vi "Get Device SN.vi"(8 "error in (no error)":errorcluster) -> (0 "error out":errorcluster, 2 "SN":string)   [LabVIEW 2018]
doc: "Returns MAC address on Windows, and device SN on RT Linux. Keeps the value in a shift register for future use."
uses:
  <vilib>/nisyscfg/nisyscfg.lvlib
  <resource>/objmgr/nisysapi.rc
  <vilib>/nisyscfg/Close (System).vi
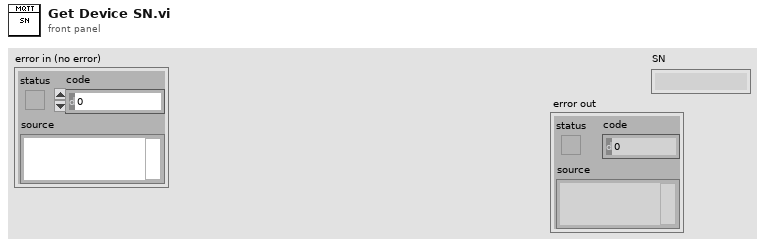
[diagram p1: front panel]
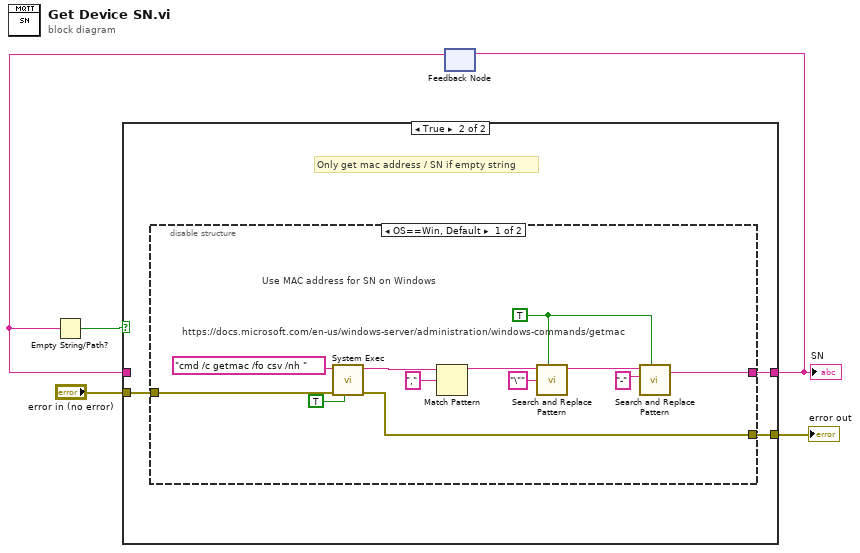
[diagram p0: block diagram]
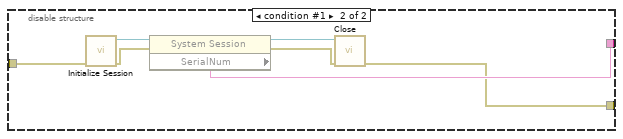
[diagram p3: hidden frame]
diagram:
  n1 = feedback #1() -> (w2:string)  [unwired: 1 in]
  n2 = Empty String/Path?(string/path=w2) -> (empty?=w1:bool)
  n3 = case shown="True" w1 {
    tunnel: [w6 w10] -> w3
    tunnel: [w7 w9] -> w5
    tunnel: "error in (no error)" -> [w7 w8]
    tunnel: w2 -> [w6 _]
    frame False {
    }
    frame True {
      # "Only get mac address / SN if empty string"
      n4 = disable-structure shown="OS==Win, Default" {
        disable-tunnel: [w13 w28] -> w10
        disable-tunnel: [w12 w24] -> w9
        disable-tunnel: w8 -> [w11 w23]
        frame condition #0 (active) {
          w15 = TRUE ("replace all? (F)")
          # "Use MAC address for SN on Windows"
          # "https://docs.microsoft.com/en-us/windows-server/administration/windows-commands/getmac"
          n5 = call <vilib>:"System Exec.vi"("run minimized? (F)"=TRUE, "error in (no error)"=w11, "command line"="cmd /c getmac /fo csv /nh ") -> ("error out"=w12:errorcluster, "standard output"=w20:string)  [unwired: 5 in, 2 out]
          n6 = Match Pattern(string=w20, regular expression="," ("delimiter (Tab)")) -> (before substring=w18:string)  [unwired: 1 in, 3 out]
          n7 = call <vilib>:"Search and Replace Pattern.vi"("string"=w18, "regular expression (\"\")"="\"" ("regular expression (\"\")"), "replace all? (F)"=w15) -> ("result string"=w14:string)  [unwired: 2 in, 1 out]
          n8 = call <vilib>:"Search and Replace Pattern.vi"("string"=w14, "regular expression (\"\")"="-" ("regular expression (\"\")"), "replace all? (F)"=w15) -> ("result string"=w13:string)  [unwired: 2 in, 1 out]
        }
        frame condition #1 {
          n9 = call <vilib>:"Initialize Session.vi"("error in (no error)"=w23) -> ("error out"=w26:errorcluster, "Session out"=w29:refnum<k21>)  [unwired: 9 in]
          n10 = property class="System Session"(reference=w29, error in=w26) -> (reference out=w27:refnum<k21>, error out=w25:errorcluster, "SerialNum"=w28:string)
          n11 = call-poly <vilib>:"Close.vi"("error in (no error)"=w25, "Session in"=w27) -> ("error out"=w24:errorcluster)  [unwired: 9 in]
        }
      }
    }
  }
  "SN" <- w3
  "error out" <- w5
  n12 = feedback-in #1(w3) -> ()
